vi "Get RIO Address.vi"(8 "error in (no error)":errorcluster, 11 "configuration file path":path) -> (0 "error out":errorcluster, 3 "RIO address out":string)   [LabVIEW 2021, in "FPGA Register IO Tests.lvclass"]
uses:
  FPGA Register IO Tests.lvclass
  <vilib>/Utility/config.llb/Read Key (String).vi
  <vilib>/Utility/config.llb/NI_LVConfig.lvlib
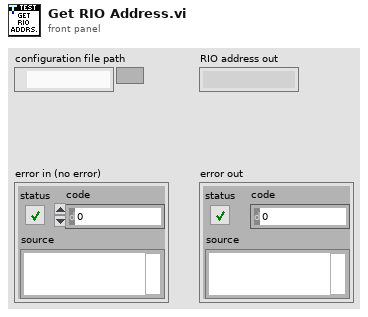
[diagram p1: front panel]
types:
  T1 = typedef "NI_LVConfig.lvlib/Config Data RefNum.ctl" = refnum<k1>
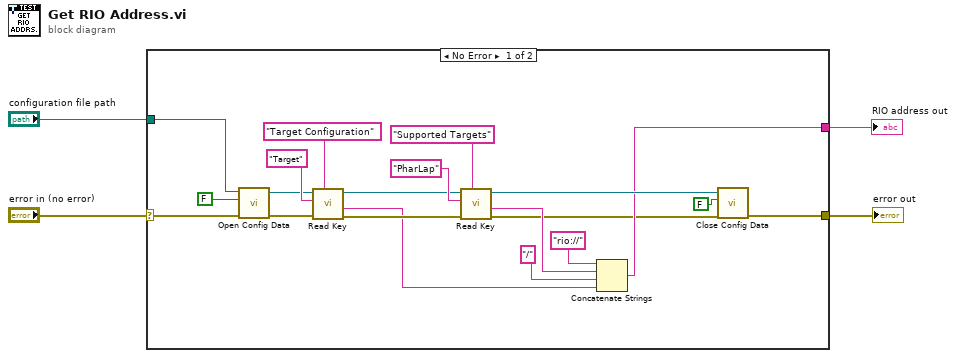
[diagram p0: block diagram]
diagram:
  n1 = case shown="No Error" "error in (no error)" {
    selector: "error in (no error)" -> [w11 w25]
    tunnel: "configuration file path" -> [w22 _]
    tunnel: [w20 w25] -> w3
    tunnel: [w6 _] -> w1
    frame No Error {
      n2 = call <vilib>:"Open Config Data.vi"("error in (no error)"=w11, "create file if necessary (T)"=FALSE, "configuration file path"=w22) -> ("error out"=w16:errorcluster, "refnum"=w15:T1)  [unwired: 6 in, 1 out]
      n3 = call-poly <vilib>:"Read Key.vi"("section"="Target Configuration", "error in (no error)"=w16, "key"="Target", "refnum"=w15) -> ("error out"=w13:errorcluster, "value"=w7:string, "refnum out"=w14:T1)  [unwired: 4 in, 1 out]
      n4 = call-poly <vilib>:"Read Key.vi"("section"="Supported Targets", "error in (no error)"=w13, "key"="PharLap", "refnum"=w14) -> ("error out"=w5:errorcluster, "value"=w9:string, "refnum out"=w12:T1)  [unwired: 4 in, 1 out]
      n5 = Concatenate Strings("rio://" ("initial string"), w9, "/" ("string"), w7) -> (w6:string)
      n6 = call <vilib>:"Close Config Data.vi"("error in (no error)"=w5, "write file if changed (T)"=FALSE, "refnum"=w12) -> ("error out"=w20:errorcluster)  [unwired: 7 in, 1 out]
    }
    frame Error {
    }
  }
  "error out" <- w3
  "RIO address out" <- w1
